vi "Read Pressure Sources.vi"(7 "Channel (0: Channel A)":enum16{"Channel A", "Channel B"}(ring), 8 "error in (no error)":errorcluster, 11 "BH Druck PACE Series in":refnum<class "BH Druck PACE Series.lvclass">) -> (0 "error out":errorcluster, 1 "Vacuum Sensor -ve Source":dbl format="%#.10g", 2 "Pressure Sensor  +ve Source":dbl format="%#.10g", 3 "BH Druck PACE Series out":refnum<class "BH Druck PACE Series.lvclass">)   [LabVIEW 2022 SP3, in "BH Druck PACE Series.lvclass"]
uses:
  BH Druck PACE Series.lvclass
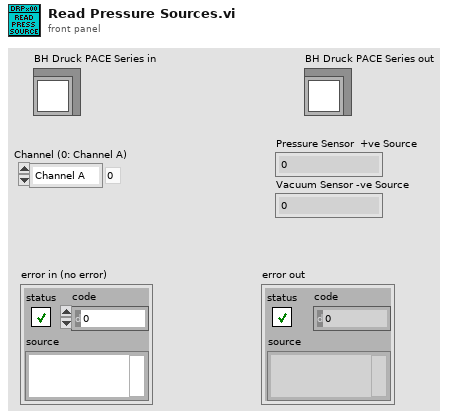
[diagram p1: front panel]
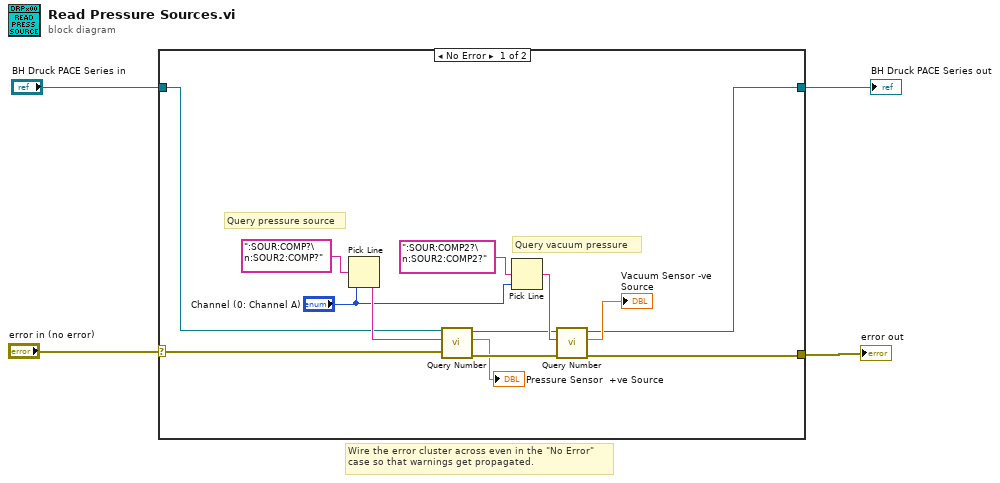
[diagram p0: block diagram]
diagram:
  # "Wire the error cluster across even in the \"No Error\"\ncase so that warnings get propagated."
  n1 = case shown="No Error" "error in (no error)" {
    selector: "error in (no error)" -> [w8 w19]
    tunnel: [w5 w19] -> w3
    tunnel: [w6 w18] -> w1
    tunnel: "BH Druck PACE Series in" -> [w7 w18]
    frame No Error {
      # "Query vacuum pressure"
      # "Query pressure source"
      n2 = Pick Line(multi-line string=":SOUR:COMP?\n:SOUR2:COMP?", line index="Channel (0: Channel A)") -> (output string=w12:string)  [unwired: 1 in]
      n3 = call-dynamic "Query Number.vi"("error in (no error)"=w8, "Query String"=w12, "BH Druck PACE Series in"=w7) -> ("error out"=w15:errorcluster, "Numeric Result"=→"Pressure Sensor  +ve Source":dbl, "BH Druck PACE Series out"=w14:refnum<class "BH Druck PACE Series.lvclass">)  [unwired: 6 in]
      n4 = Pick Line(multi-line string=":SOUR:COMP2?\n:SOUR2:COMP2?", line index="Channel (0: Channel A)") -> (output string=w17:string)  [unwired: 1 in]
      n5 = call-dynamic "Query Number.vi"("error in (no error)"=w15, "Query String"=w17, "BH Druck PACE Series in"=w14) -> ("error out"=w5:errorcluster, "Numeric Result"=→"Vacuum Sensor -ve Source":dbl, "BH Druck PACE Series out"=w6:refnum<class "BH Druck PACE Series.lvclass">)  [unwired: 6 in]
    }
    frame Error {
    }
  }
  "error out" <- w3
  "BH Druck PACE Series out" <- w1
